vi "Process.vi"(8 "error in (no error)":errorcluster, 10 "Pound in":refnum<class "Pound.lvclass">, 11 "Qbus in":refnum<class "Qbus.lvclass">) -> (0 "error out":errorcluster)   [LabVIEW 2017, in "ScanEngine.lvlib"]
doc: "This process acquires data from channels on modules whose sampling mode property is single-point. These channels acquire a single value per read instead of continuously acquiring samples at a high sampling rate. In other words, this process does not acquire data as waveforms. This process relies on the NI Scan Engine interface rather than the FPGA interface, which means it reads and updates all single-point values at a one-second sample rate."
uses:
  <vilib>/addons/InsightCM/Devices/Shared/Common/ScanEngine/ScanEngine.lvlib
  <vilib>/addons/Qbus/Qbus.lvclass
  <vilib>/NI/Software Watchdog/Pound/Pound.lvclass
  <vilib>/addons/InsightCM/Devices/Shared/Common/ScanEngine/controls/Configuration.ctl
  <vilib>/addons/InsightCM/Devices/Shared/Common/ScanEngine/controls/Group.ctl
  <vilib>/addons/InsightCM/Devices/Shared/Common/ScanEngine/controls/Channel.ctl
  <vilib>/Utility/Data Type/Type Definitions/Data Type.ctl
  <vilib>/addons/InsightCM/MessageBus/Base/controls/KeyValuePair.ctl
  <vilib>/addons/TimerProcess/controls/taskType.ctl
  <vilib>/NI/Software Watchdog/Watchdog/Watchdog.lvclass
  <vilib>/addons/TraceLogger/TraceLogger.lvlib
  <vilib>/addons/TimerProcess/TimerProcess.lvlib
  <vilib>/addons/InsightCM/Devices/Shared/Common/FpgaBitfileManager/FpgaBitfileManager.lvlib
  <vilib>/addons/InsightCM/Utilities/GlobalConfiguration/GlobalConfiguration.lvlib
  <vilib>/addons/InsightCM/Devices/Shared/Common/ServerComm/ServerComm.lvlib
  <vilib>/Utility/Data Type/NI_Data Type.lvlib
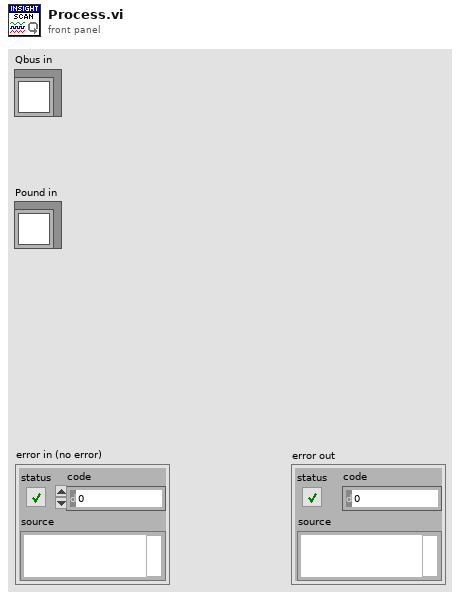
[diagram p1: front panel]
types:
  T1 = typedef "ScanEngine.lvlib/Configuration.ctl" = cluster{"DynamicFPGAVIRef":refnum<k20>, "Device":string, "Groups":T2[]}
  T2 = typedef "ScanEngine.lvlib/Group.ctl" = cluster{"Group":string, "Channels":T3[]}
  T3 = typedef "ScanEngine.lvlib/Channel.ctl" = cluster{"Name":string, "Hardware Channel":string, "ChannelType":string, "TrendPoint Id":string, "Value":sgl, "Slope":dbl, "Offset":dbl, "IO variable":refnum<k21>, "datatype":T4, "Properties":T5[]}
  T4 = typedef "NI_Data Type.lvlib/Data Type.ctl" = enum8{"Invalid Type", "Void", "I8", "I16", "I32", "I64", "U8", "U16", "U32", "U64", "Single Float", "Double Float", "Extended Float", "Single Complex", "Double Complex", "Extended Complex", "Enum U8", "Enum U16", "Enum U32", "Enum U64", "Single Float With Unit", "Double Float With Unit", "Extended Float With Unit", "Single Complex with Unit", "Double Complex with Unit", "Extended Complex with Unit", "Boolean", "String", "Path", "Picture", "Tag", "Array", "Cluster", "Variant", "LV Variant", "Waveform", "Timestamp", "Digital Waveform", "Digital Data", "ExpressData", "Refnum", "External Data", "VI", "Poly VI", "LabVIEW Class Instance", "Fixed Point"}
  T5 = typedef "KeyValuePair.ctl" = cluster{"Key":string, "Value":string}
  T6 = typedef "TimerProcess.lvlib/taskType.ctl" = enum16{"single", "repeat"}
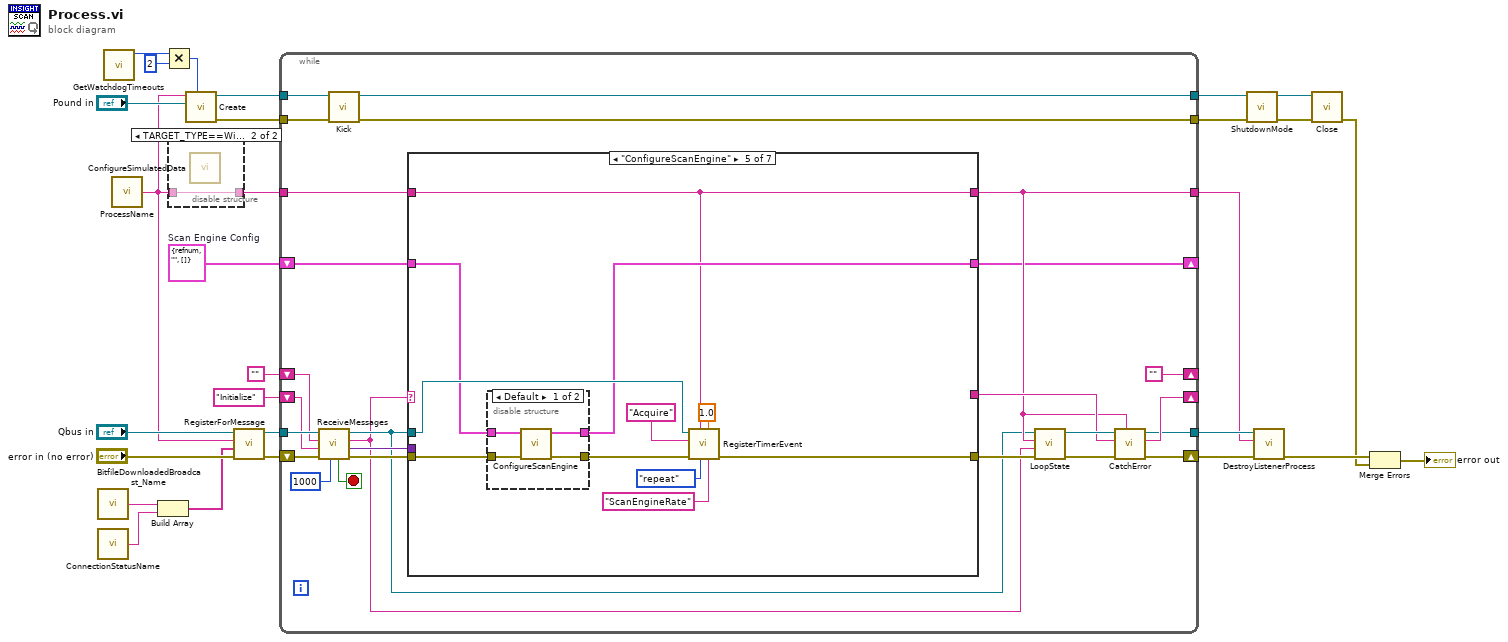
[diagram p0: block diagram]
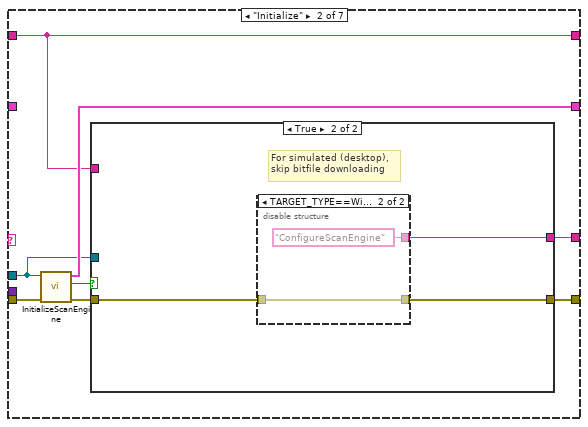
[diagram p4: hidden frame]
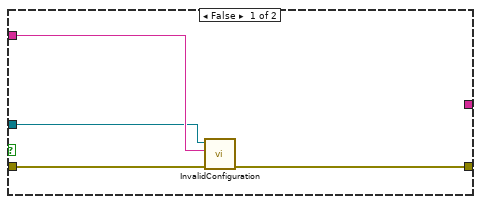
[diagram p5: hidden frame]
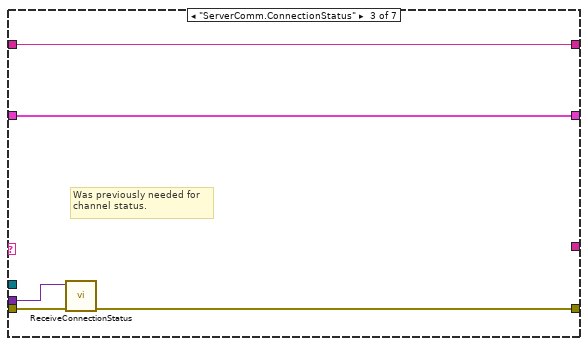
[diagram p7: hidden frame]
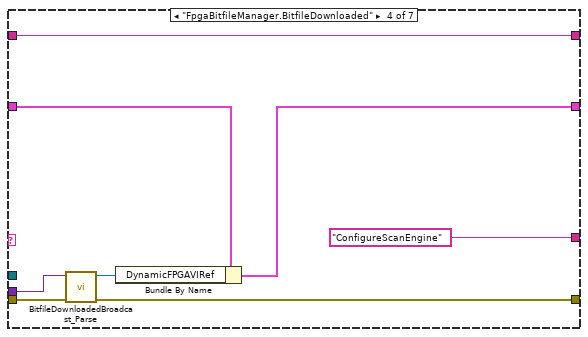
[diagram p8: hidden frame]
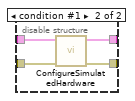
[diagram p9: hidden frame]
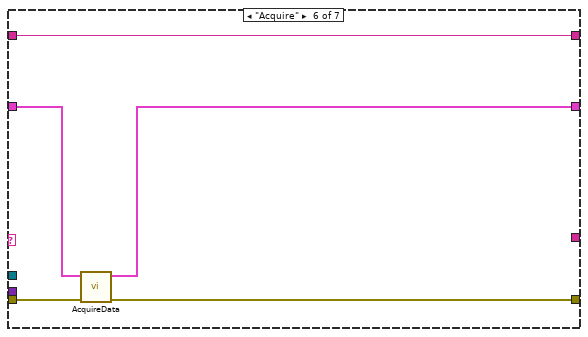
[diagram p10: hidden frame]
diagram:
  w13 = T1 {"DynamicFPGAVIRef"=refnum, "Device"="", "Groups"=[]}  # Scan Engine Config
  n1 = call <vilib>:"BitfileDownloadedBroadcast_Name.vi"() -> ("message name"=w7:string)  [unwired: 5 in]
  n2 = call <vilib>:"ConnectionStatusName.vi"() -> ("message name"=w6:string)  [unwired: 5 in]
  n3 = call <vilib>:"GetWatchdogTimeouts.vi"() -> ("software timeout"=w3:u32)  [unwired: 10 in, 1 out]
  n4 = call <vilib>:"ProcessName.vi"() -> ("ProcessName"=w4:string)  [unwired: 5 in]
  n5 = Build Array(w7, w6) -> (w8:string[])
  n6 = Multiply(x=w3, y=u32 2) -> (x*y=w1:u32)
  n7 = disable-structure shown="TARGET_TYPE==Windows" {
    disable-tunnel: [w29 w30] -> w5
    disable-tunnel: w4 -> [w29 w30]
    frame condition #0 (active) {
    }
    frame condition #1 {
      n8 = call <vilib>:"ConfigureSimulatedData.vi"() -> ()  [unwired: 11 in, 1 out]
    }
  }
  n9 = call <vilib>:"Create.vi"("Execution Timeout (ms)"=w1, "Pound"="Pound in", "Name"=w4) -> ("error out"=w25:errorcluster, "Watchdog"=w26:refnum<data-value>)  [unwired: 7 in]
  n10 = call <vilib>:"RegisterForMessage.vi"("error in (no error)"="error in (no error)", "message names"=w8, "process name"=w4, "Qbus in"="Qbus in") -> ("error in (no error)"=w9:errorcluster, "Qbus out"=w10:refnum<class "Qbus.lvclass">)  [unwired: 6 in]
  n11 = while {
    shift-right: [""] -> _
    shift-left: "" -> [w54]
    tunnel: w5 -> [w40]
    shift-right: [w43] -> _
    shift-left: "Initialize" -> [w53]
    tunnel: w10 -> [w55]
    tunnel: w26 -> [w52]
    tunnel: w25 -> [w51]
    tunnel: [w49] -> w22
    tunnel: [w48] -> w21
    tunnel: [w41] -> w18
    tunnel: [w39] -> w17
    shift-right: [w36] -> _
    shift-left: w13 -> [w35]
    shift-right: [w42] -> w19
    shift-left: w9 -> [w56]
    stop <- w34 stop-if-true
    n12 = call <vilib>:"ReceiveMessages.vi"("Timeout(100)"=1000 ("milliseconds to wait"), "error in (no error)"=w56, "Priority Action"=w53, "Default Action"=w54, "Qbus in"=w55) -> ("error out"=w50:errorcluster, "MsgValue"=w38:variant, "Action"=w33:string, "Qbus out"=w37:refnum<class "Qbus.lvclass">, "exit"=w34:bool)  [unwired: 2 in]
    n13 = call <vilib>:"Kick.vi"("error in (no error)"=w51, "Watchdog"=w52) -> ("error out"=w48:errorcluster, "Watchdog"=w49:refnum<data-value>)  [unwired: 8 in]
    n14 = case shown="\"ConfigureScanEngine\"" w33 {
      tunnel: w50 -> [w59 w67 w81 w87 w101 w114 w115]
      tunnel: [w59 w64 w80 w84 w91 w112 w115] -> w46
      tunnel: w37 -> [_ w61 _ _ w100 _ _]
      tunnel: [_ w66 _ "ConfigureScanEngine" _ _ _] -> w44
      tunnel: w38 -> [_ _ w79 w86 _ _ _]
      tunnel: w40 -> [w58 w62 w82 w90 w92 w113 w116]
      tunnel: [w58 w62 w82 w90 w92 w113 w116] -> w39
      tunnel: w35 -> [w57 _ w78 w89 w94 w111 w117]
      tunnel: [w57 w63 w78 w88 w93 w110 w117] -> w36
      frame Default {
        (unwired) 100
      }
      frame "Initialize" {
        n15 = call <vilib>:"InitializeScanEngine.vi"("error in (no error)"=w67, "Qbus"=w61) -> ("error out"=w65:errorcluster, "valid"=w60:bool, "scan engine config"=w63:T1)  [unwired: 7 in]
        n16 = case shown="True" w60 {
          tunnel: w61 -> [w69 _]
          tunnel: [_ w74] -> w66
          tunnel: w65 -> [w68 w72]
          tunnel: [w71 w73] -> w64
          tunnel: w62 -> [w70 _]
          frame False {
            n17 = call <vilib>:"InvalidConfiguration.vi"("error in (no error)"=w68, "description"=w70, "Qbus in"=w69) -> ("error out"=w71:errorcluster)  [unwired: 7 in, 1 out]
          }
          frame True {
            # "For simulated (desktop),\nskip bitfile downloading"
            n18 = disable-structure shown="TARGET_TYPE==Windows||OS==VxWorks" {
              disable-tunnel: w72 -> [w75 w76]
              disable-tunnel: [w75 w76] -> w73
              disable-tunnel: [_ "ConfigureScanEngine"] -> w74
              frame condition #0 (active) {
              }
              frame condition #1 {
              }
            }
          }
        }
      }
      frame "ServerComm.ConnectionStatus" {
        # "Was previously needed for\nchannel status."
        n19 = call <vilib>:"ReceiveConnectionStatus.vi"("error in (no error)"=w81, "body"=w79) -> ("error out"=w80:errorcluster)  [unwired: 6 in, 3 out]
      }
      frame "FpgaBitfileManager.BitfileDownloaded" {
        n20 = call <vilib>:"BitfileDownloadedBroadcast_Parse.vi"("error in (no error)"=w87, "data"=w86) -> ("error out"=w84:errorcluster, "FPGA reference"=w85:refnum<k20>)  [unwired: 8 in]
        n21 = Bundle By Name(cluster=w89, "DynamicFPGAVIRef"=w85) -> (w88:T1)
      }
      frame "ConfigureScanEngine" {
        n22 = disable-structure shown="Default" {
          disable-tunnel: w94 -> [w103 w109]
          disable-tunnel: [w102 w108] -> w93
          disable-tunnel: w101 -> [w105 w107]
          disable-tunnel: [w104 w106] -> w95
          frame condition #0 (active) {
            n23 = call <vilib>:"ConfigureScanEngine.vi"("error in (no error)"=w105, "Scan Engine Config"=w103) -> ("error out"=w104:errorcluster, "Scan Engine Config out"=w102:T1)  [unwired: 8 in]
          }
          frame condition #1 {
            n24 = call <vilib>:"ConfigureSimulatedHardware.vi"("error in (no error)"=w107, "Scan Engine Config"=w109) -> ("error out"=w106:errorcluster, "Scan Engine Config Out"=w108:T1)  [unwired: 8 in]
          }
        }
        n25 = call <vilib>:"RegisterTimerEvent.vi"("timer task name"="ScanEngineRate" ("Name"), "interval (sec)"=1.0, "type"=taskType."repeat", "process name"=w92, "error in (no error)"=w95, "callback action"="Acquire", "qbus in"=w100) -> ("error out"=w91:errorcluster)  [unwired: 3 in, 1 out]
      }
      frame "Acquire" {
        n26 = call <vilib>:"AcquireData.vi"("error in (no error)"=w114, "config in"=w111) -> ("error out"=w112:errorcluster, "config out"=w110:T1)  [unwired: 8 in]
      }
      frame "Exit" {
      }
    }
    n27 = call <vilib>:"LoopState.vi"("error in (no error)"=w46, "loop action"=w33, "process name"=w39, "Qbus in"=w37) -> ("error out"=w45:errorcluster, "Qbus out"=w47:refnum<class "Qbus.lvclass">)  [unwired: 6 in]
    n28 = call <vilib>:"CatchError.vi"("source"=w39, "error in (no error)"=w45, "next action in"=w44, "Qbus in"=w47) -> ("error out"=w42:errorcluster, "next action out"=w43:string, "Qbus out"=w41:refnum<class "Qbus.lvclass">)  [unwired: 5 in]
  }
  n29 = call <vilib>:"ShutdownMode.vi"("error in (no error)"=w21, "Watchdog"=w22) -> ("error out"=w23:errorcluster, "Watchdog"=w24:refnum<data-value>)  [unwired: 8 in]
  n30 = call <vilib>:"DestroyListenerProcess.vi"("error in (no error)"=w19, "process name"=w17, "Qbus in"=w18) -> ("error in (no error)"=w16:errorcluster)  [unwired: 7 in, 1 out]
  n31 = call <vilib>:"Close.vi"("error in (no error)"=w23, "Watchdog"=w24) -> ("error out"=w15:errorcluster)  [unwired: 9 in]
  n32 = Merge Errors(w16, w15) -> (→"error out":errorcluster)
